vi "Configure Waveform Trigger Source.vi"(8 "error in (no error)":errorcluster {"code" format="%.0x"}, 9 "Source (2: Immediate)":u16(ring)=2 items=["External", "Software", "Immediate"], 11 "VISA resource name":refnum<visa-resource-name>) -> (0 "error out":errorcluster {"code" format="%.0x"}, 3 "VISA resource name out":refnum<visa-resource-name>)   [LabVIEW 2014, in "Agilent N6700 Series.lvlib"]
doc: "Configures the trigger source of the waveform.\n\n<b>Note:</b>\nThis VI only applies to the N6705B and N6705C DC Power Analyzer."
uses:
  Agilent N6700 Series.lvlib
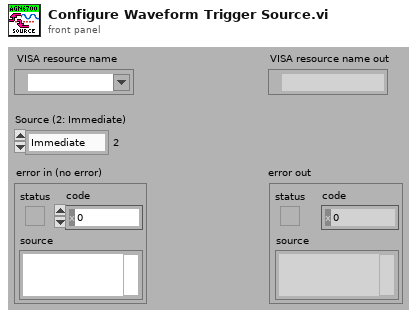
[diagram p1: front panel]
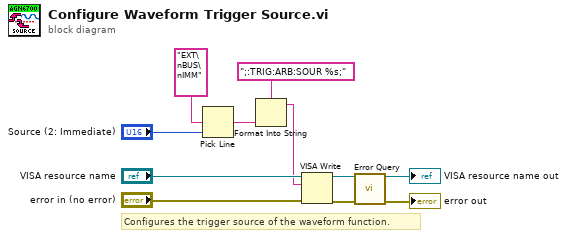
[diagram p0: block diagram]
diagram:
  # "Configures the trigger source of the waveform function."
  n1 = Pick Line(multi-line string="EXT\nBUS\nIMM", line index="Source (2: Immediate)") -> (output string=w7:string)  [unwired: 1 in]
  n2 = Format Into String(format string=";:TRIG:ARB:SOUR %s;", w7) -> (resulting string=w5:string)  [unwired: 2 in, 1 out]
  n3 = VISA Write(VISA resource name="VISA resource name", write buffer=w5, error in (no error)="error in (no error)") -> (VISA resource name out=w2:refnum<visa-resource-name>, error out=w1:errorcluster)  [unwired: 1 out]
  n4 = call "Error Query.vi"("VISA resource name"=w2, "error in (no error)"=w1) -> ("VISA resource name out"=→"VISA resource name out":refnum<visa-resource-name>, "error out"=→"error out":errorcluster)  [unwired: 10 in, 2 out]
